vi "Read Fault Event.vi"(8 "error in (no error)":errorcluster, 11 "Fault_Engine in":refnum<class "Engine.lvclass">) -> (0 "error out":errorcluster, 2 "Fault event":refnum<user-event>, 3 "Fault_Engine out":refnum<class "Engine.lvclass">)   [LabVIEW 2019, in "Engine.lvlib" / "Engine.lvclass"]
uses:
  Project/Engine.lvclass
  Project/Engine.lvclass/Engine.ctl
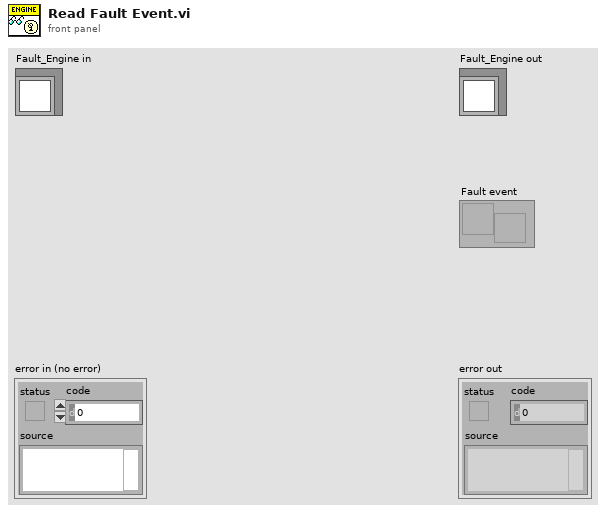
[diagram p1: front panel]
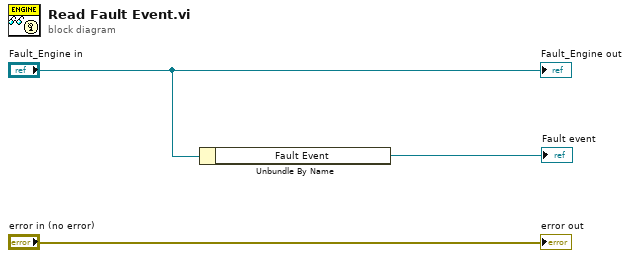
[diagram p0: block diagram]
diagram:
  n1 = Unbundle By Name("Fault_Engine in") -> ("Fault Event"=→"Fault event":refnum<user-event>)
  "error out" <- "error in (no error)"
  "Fault_Engine out" <- "Fault_Engine in"
